vi "VISA - Open Connection.vi"(7 "Enable Termination\nChar (T)":bool, 8 "error in":errorcluster, 11 "VISA resource name":refnum<visa-resource-name>="COM6") -> (0 "error out":errorcluster, 3 "VISA Ref":refnum<visa-resource-name>)   [LabVIEW 2019]
uses:
  <vilib>/Instr/_visa.llb/VISA Flush IO Buffer Mask.ctl
  <vilib>/Instr/_visa.llb/VISA Configure Serial Port (Instr).vi
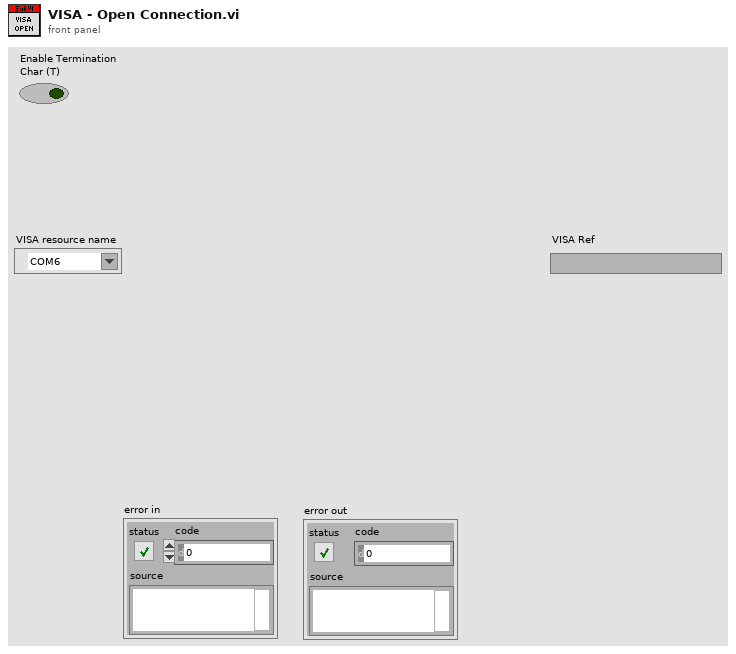
[diagram p1: front panel]
types:
  T1 = typedef "VISA Flush IO Buffer Mask.ctl" = u16
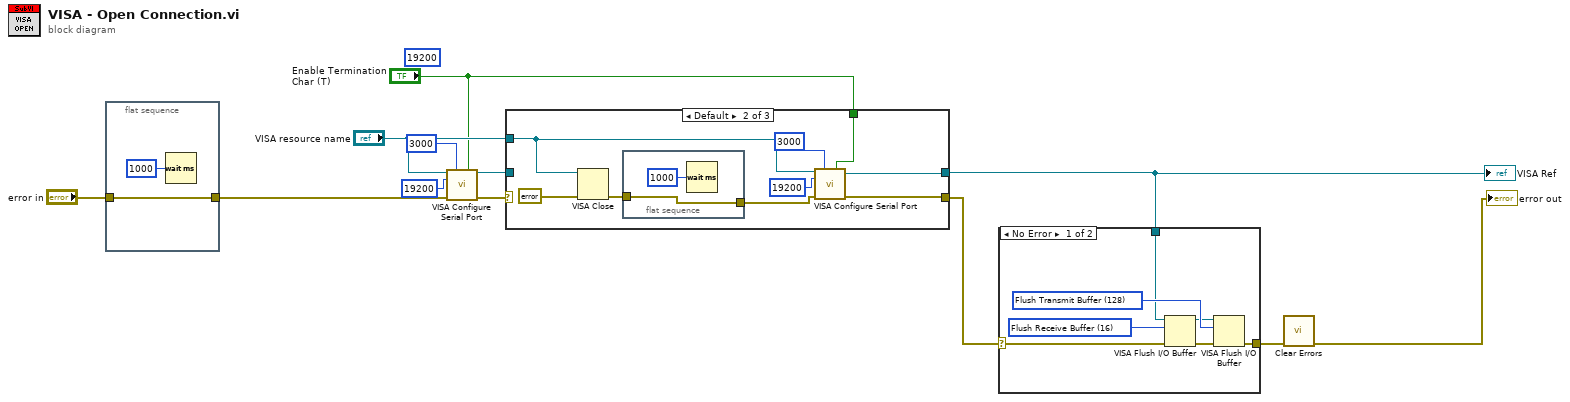
[diagram p0: block diagram]
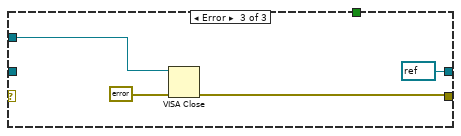
[diagram p4: hidden frame]
diagram:
  (unwired) u32 19200 ("baud rate (9600)")
  n1 = flat-sequence {
    tunnel: [w13] -> w2
    tunnel: "error in" -> [w13]
    frame #0 {
      n2 = Wait (ms)(milliseconds to wait=u32 1000) -> ()  [unwired: 1 out]
    }
  }
  n3 = call-poly "VISA Configure Serial Port"("VISA resource name"="VISA resource name", "timeout (10sec)"=u32 3000, "Enable Termination\nChar (T)"="Enable Termination\nChar (T)", "baud rate (9600)"=u32 19200, "error in (no error)"=w2) -> ("VISA resource name out"=w10:refnum<visa-resource-name>, "error out"=w11:errorcluster)  [unwired: 9 in]
  n4 = case shown="Default" w11 {
    selector: w11 -> [w15 _ _]
    tunnel: [w16 w22 refnum<visa-resource-name> refnum ("VISA resource name out")] -> w5
    tunnel: w10 -> [w16 _ _]
    tunnel: [w15 w21 w29] -> w7
    tunnel: "VISA resource name" -> [_ w23 w30]
    tunnel: "Enable Termination\nChar (T)" -> [_ w19 _]
    frame No Error {
    }
    frame Default {
      n5 = VISA Close(VISA resource name=w23, error in (no error)=errorcluster {"status"=FALSE, "code"=0, "source"=""} ("error IO")) -> (error out=w17:errorcluster)
      n6 = flat-sequence {
        tunnel: [w26] -> w18
        tunnel: w17 -> [w26]
        frame #0 {
          n7 = Wait (ms)(milliseconds to wait=u32 1000) -> ()  [unwired: 1 out]
        }
      }
      n8 = call-poly "VISA Configure Serial Port"("VISA resource name"=w23, "timeout (10sec)"=u32 3000, "Enable Termination\nChar (T)"=w19, "baud rate (9600)"=u32 19200, "error in (no error)"=w18) -> ("VISA resource name out"=w22:refnum<visa-resource-name>, "error out"=w21:errorcluster)  [unwired: 9 in]
    }
    frame Error {
      n9 = VISA Close(VISA resource name=w30, error in (no error)=errorcluster {"status"=FALSE, "code"=0, "source"=""} ("error IO")) -> (error out=w29:errorcluster)
    }
  }
  "VISA Ref" <- w5
  n10 = case shown="No Error" w7 {
    selector: w7 -> [w32 w39]
    tunnel: [w34 w39] -> w6
    tunnel: w5 -> [w33 _]
    frame No Error {
      w37 = T1 128 items=["Flush Receive Buffer"=16, "Write Transmit Buffer to Device"=32, "Flush Receive Buffer (No I/O)"=64, "Flush Transmit Buffer"=128] ("Mask")
      w38 = T1 16 items=["Flush Receive Buffer"=16, "Write Transmit Buffer to Device"=32, "Flush Receive Buffer (No I/O)"=64, "Flush Transmit Buffer"=128] ("Mask")
      n11 = VISA Flush I/O Buffer(VISA resource name=w33, mask (16)=w38, error in (no error)=w32) -> (VISA resource name out=w35:refnum<visa-resource-name>, error out=w36:errorcluster)
      n12 = VISA Flush I/O Buffer(VISA resource name=w35, mask (16)=w37, error in (no error)=w36) -> (error out=w34:errorcluster)  [unwired: 1 out]
    }
    frame Error {
    }
  }
  n13 = call <vilib>:"Clear Errors.vi"("error in (no error)"=w6) -> ("error out"=→"error out":errorcluster)  [unwired: 5 in, 1 out]
